vi "hahn plus RF rabi.vi"(3 "MW Delay":dbl, 4 "Pulse offset":dbl, 5 "Tau":dbl, 6 "RF tau Stop":dbl=1.0 format="%0.2f", 7 "Rabi Frequency":dbl, 8 "RF tau Start":dbl format="%0.2f", 9 "RF tau # samples":i32=128, 10 "No. Instructions":i32, 11 "Optical Pulse":T1(array[cluster])) -> (0 "Pulse Sequence":T1(array[cluster]), 1 "Array":dbl[](array[numeric]))   [LabVIEW 2012]
uses:
  <vilib>/Analysis/1siggen.llb/Ramp Pattern by Samples.vi
  <vilib>/Analysis/NI_AALBase.lvlib
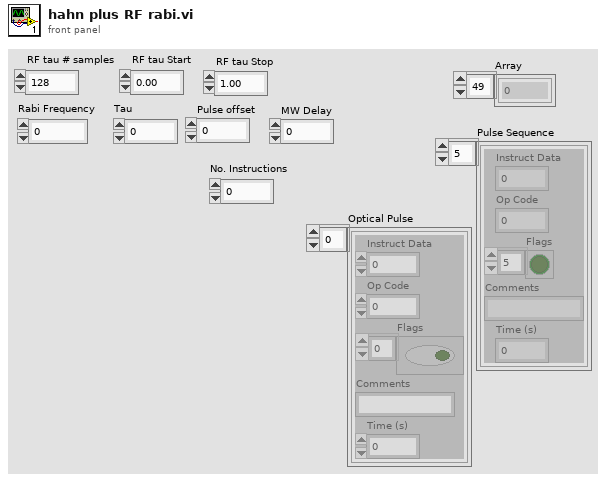
[diagram p1: front panel]
types:
  T1 = cluster{"Instruct Data":i32, "Op Code":i32, "Flags":bool[], "Comments":string, "Time (s)":dbl}[]
  T2 = cluster{"Instruct Data":i32, "Op Code":i32, "Flags":bool[], "Comments":string, "Time (s)":dbl}
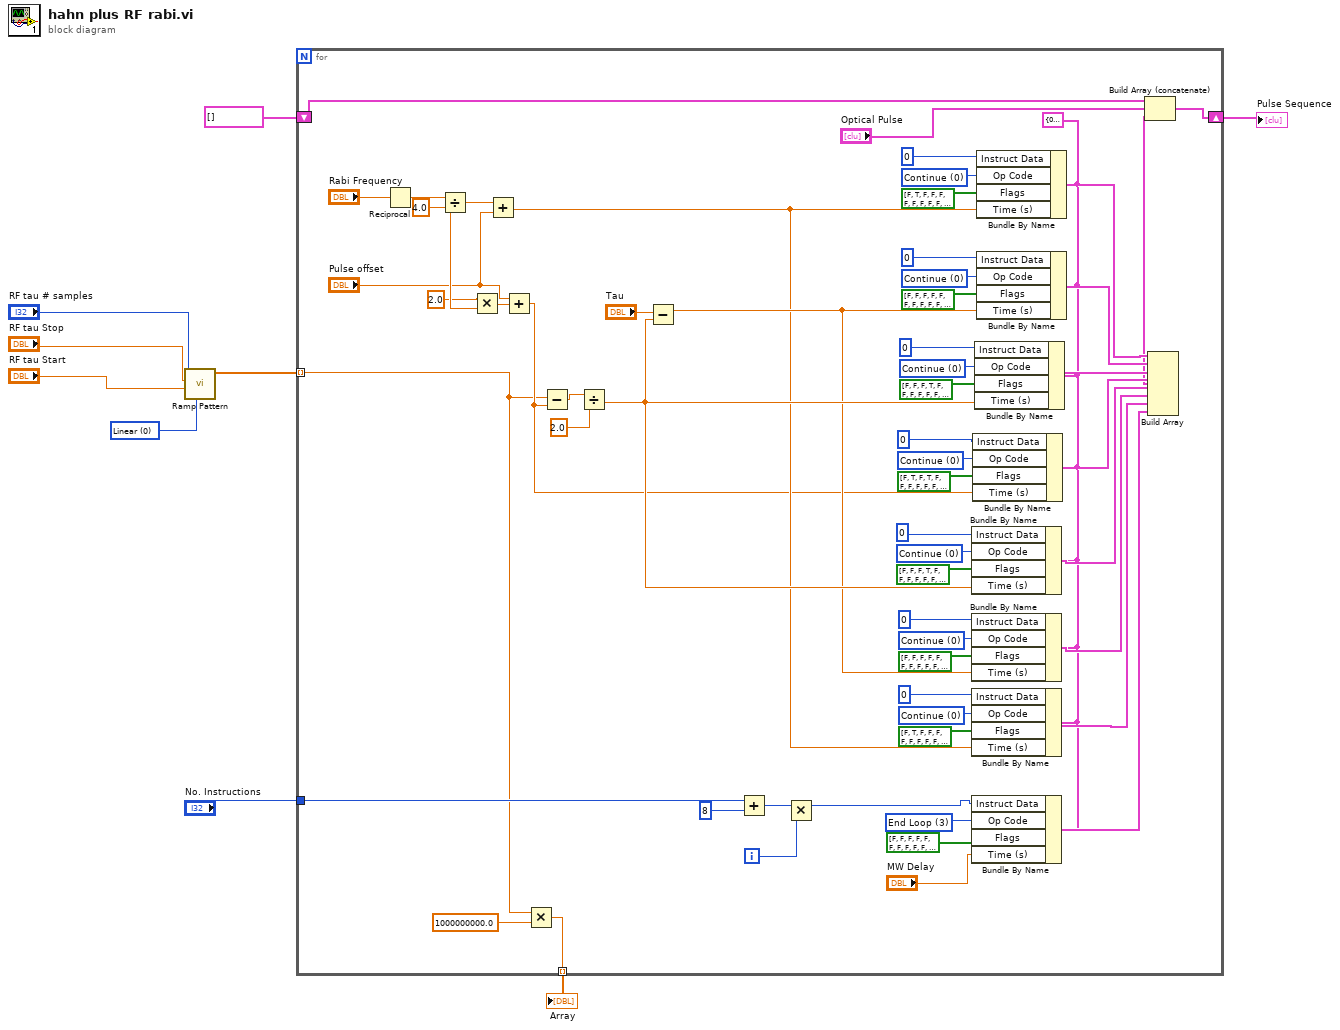
[diagram p0: block diagram]
diagram:
  w5 = u16 0 items=["Linear", "Logarithmic"] ("type")
  n1 = call-poly <vilib>:"Ramp Pattern.vi"("type"=w5, "start"="RF tau Start", "end"="RF tau Stop", "samples"="RF tau # samples") -> ("Ramp Pattern"=w9:dbl[])  [unwired: 6 in, 1 out]
  n2 = for {
    tunnel: w9 -> [w13] mode=indexing
    tunnel: "No. Instructions" -> [w20]
    shift-right: [w14] -> w2
    shift-left: T1 [] -> [w10]
    tunnel: [w11] -> w1 mode=indexing
    i -> [w17]
    w36 = 0 items=["Continue", "Stop", "Loop", "End Loop", "JSR", "RTS", "Branch", "Long Delay", "Wait"] ("Op Code")
    w39 = 0 items=["Continue", "Stop", "Loop", "End Loop", "JSR", "RTS", "Branch", "Long Delay", "Wait"] ("Op Code")
    w47 = 0 items=["Continue", "Stop", "Loop", "End Loop", "JSR", "RTS", "Branch", "Long Delay", "Wait"] ("Op Code")
    w50 = 0 items=["Continue", "Stop", "Loop", "End Loop", "JSR", "RTS", "Branch", "Long Delay", "Wait"] ("Op Code")
    w54 = 0 items=["Continue", "Stop", "Loop", "End Loop", "JSR", "RTS", "Branch", "Long Delay", "Wait"] ("Op Code")
    w57 = 0 items=["Continue", "Stop", "Loop", "End Loop", "JSR", "RTS", "Branch", "Long Delay", "Wait"] ("Op Code")
    w60 = 0 items=["Continue", "Stop", "Loop", "End Loop", "JSR", "RTS", "Branch", "Long Delay", "Wait"] ("Op Code")
    w67 = 3 items=["Continue", "Stop", "Loop", "End Loop", "JSR", "RTS", "Branch", "Long Delay", "Wait"] ("Op Code")
    w23 = T2 {"Instruct Data"=0, "Op Code"=0, "Flags"=[FALSE, FALSE, FALSE, FALSE, FALSE, FALSE, FALSE, FALSE, FALSE, FALSE, FALSE, FALSE, FALSE, FALSE, FALSE, FALSE, FALSE, FALSE, FALSE, FALSE, FALSE, TRUE, TRUE, TRUE], "Comments"="", "Time (s)"=0.01} ("PB Inst 2")
    n3 = Reciprocal(x="Rabi Frequency") -> (1/x=w65:dbl)
    n4 = Divide(x=w65, y=4.0) -> (x/y=w64:dbl)
    n5 = Multiply(x=2.0, y=w64) -> (x*y=w52:dbl)
    n6 = Add(x=w64, y="Pulse offset") -> (x+y=w26:dbl)
    n7 = Add(x="Pulse offset", y=w52) -> (x+y=w25:dbl)
    n8 = Multiply(x=w13, y=1000000000.0) -> (x*y=w11:dbl)
    n9 = Subtract(x=w13, y=w25) -> (x-y=w44:dbl)
    n10 = Divide(x=w44, y=2.0) -> (x/y=w41:dbl)
    n11 = Subtract(x="Tau", y=w41) -> (x-y=w34:dbl)
    n12 = Add(x=w20, y=8) -> (x+y=w21:i32)
    n13 = Multiply(x=w21, y=w17) -> (x*y=w18:i32)
    n14 = Bundle By Name(cluster=w23, "Instruct Data"=0, "Op Code"=w47, "Flags"=bool[] [FALSE, FALSE, FALSE, TRUE, FALSE, FALSE, FALSE, FALSE, FALSE, FALSE, FALSE, FALSE, FALSE, FALSE, FALSE, FALSE, FALSE, FALSE, FALSE, FALSE, FALSE, TRUE, TRUE, TRUE], "Time (s)"=w41) -> (w29:T2)
    n15 = Bundle By Name(cluster=w23, "Instruct Data"=0, "Op Code"=w39, "Flags"=bool[] [FALSE, FALSE, FALSE, FALSE, FALSE, FALSE, FALSE, FALSE, FALSE, FALSE, FALSE, FALSE, FALSE, FALSE, FALSE, FALSE, FALSE, FALSE, FALSE, FALSE, FALSE, TRUE, TRUE, TRUE], "Time (s)"=w34) -> (w28:T2)
    n16 = Bundle By Name(cluster=w23, "Instruct Data"=0, "Op Code"=w36, "Flags"=bool[] [FALSE, TRUE, FALSE, FALSE, FALSE, FALSE, FALSE, FALSE, FALSE, FALSE, FALSE, FALSE, FALSE, FALSE, FALSE, FALSE, FALSE, FALSE, FALSE, FALSE, FALSE, TRUE, TRUE, TRUE], "Time (s)"=w26) -> (w27:T2)
    n17 = Bundle By Name(cluster=w23, "Instruct Data"=w18, "Op Code"=w67, "Flags"=bool[] [FALSE, FALSE, FALSE, FALSE, FALSE, FALSE, FALSE, FALSE, FALSE, FALSE, FALSE, FALSE, FALSE, FALSE, FALSE, FALSE, FALSE, FALSE, FALSE, FALSE, FALSE, TRUE, TRUE, TRUE], "Time (s)"="MW Delay") -> (w24:T2)
    n18 = Bundle By Name(cluster=w23, "Instruct Data"=0, "Op Code"=w50, "Flags"=bool[] [FALSE, TRUE, FALSE, TRUE, FALSE, FALSE, FALSE, FALSE, FALSE, FALSE, FALSE, FALSE, FALSE, FALSE, FALSE, FALSE, FALSE, FALSE, FALSE, FALSE, FALSE, TRUE, TRUE, TRUE], "Time (s)"=w25) -> (w30:T2)
    n19 = Bundle By Name(cluster=w23, "Instruct Data"=0, "Op Code"=w54, "Flags"=bool[] [FALSE, FALSE, FALSE, TRUE, FALSE, FALSE, FALSE, FALSE, FALSE, FALSE, FALSE, FALSE, FALSE, FALSE, FALSE, FALSE, FALSE, FALSE, FALSE, FALSE, FALSE, TRUE, TRUE, TRUE], "Time (s)"=w41) -> (w31:T2)
    n20 = Bundle By Name(cluster=w23, "Instruct Data"=0, "Op Code"=w60, "Flags"=bool[] [FALSE, TRUE, FALSE, FALSE, FALSE, FALSE, FALSE, FALSE, FALSE, FALSE, FALSE, FALSE, FALSE, FALSE, FALSE, FALSE, FALSE, FALSE, FALSE, FALSE, FALSE, TRUE, TRUE, TRUE], "Time (s)"=w26) -> (w33:T2)
    n21 = Bundle By Name(cluster=w23, "Instruct Data"=0, "Op Code"=w57, "Flags"=bool[] [FALSE, FALSE, FALSE, FALSE, FALSE, FALSE, FALSE, FALSE, FALSE, FALSE, FALSE, FALSE, FALSE, FALSE, FALSE, FALSE, FALSE, FALSE, FALSE, FALSE, FALSE, TRUE, TRUE, TRUE], "Time (s)"=w34) -> (w32:T2)
    n22 = Build Array(w33, w32, w31, w30, w29, w28, w27, w24) -> (w16:T1)
    n23 = Build Array (concatenate)(w10, "Optical Pulse", w16) -> (w14:T1)
  }
  "Pulse Sequence" <- w2
  "Array" <- w1
